vi "获取MPPT状态.vi"(8 "error in (no error)":errorcluster, 11 "MB session in":refnum<class "MB_Master.lvclass">) -> (0 "error out":errorcluster, 1 "结果字符串":string caption="状态", 2 "状态":T1, 3 "MB session out":refnum<class "MB_Master.lvclass">)   [LabVIEW 2016, in "环境动力单元.lvlib"]
uses:
  <vilib>/Plasmionique/MB Master/MB_Master/MB_Master.lvclass
  <vilib>/Plasmionique/MB Master/MB Master.lvlib
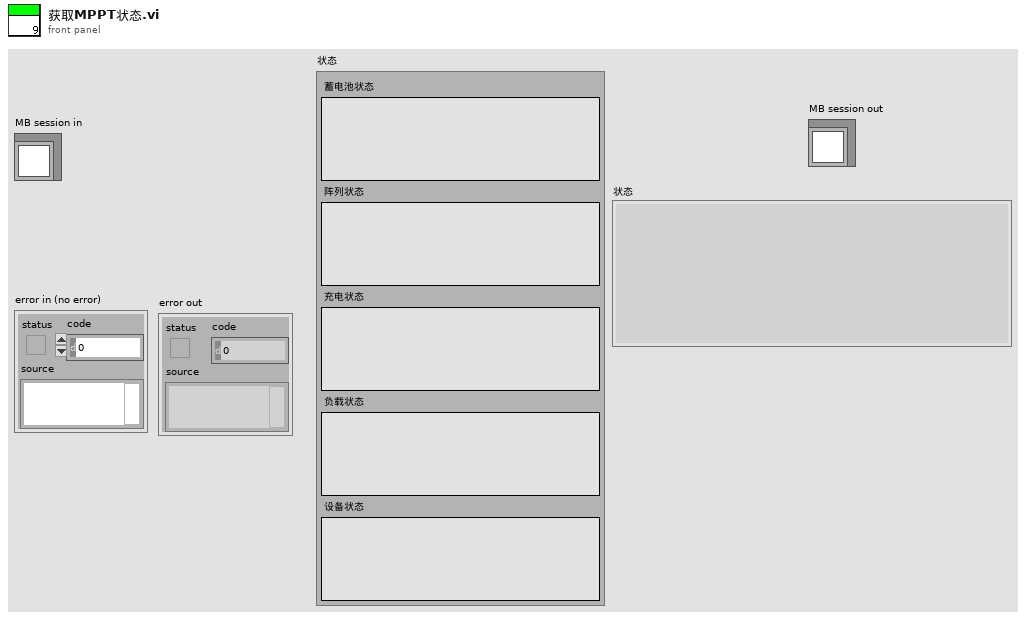
[diagram p1: front panel]
types:
  T1 = cluster{"蓄电池状态":string, "阵列状态":string, "充电状态":string, "负载状态":string, "设备状态":string}
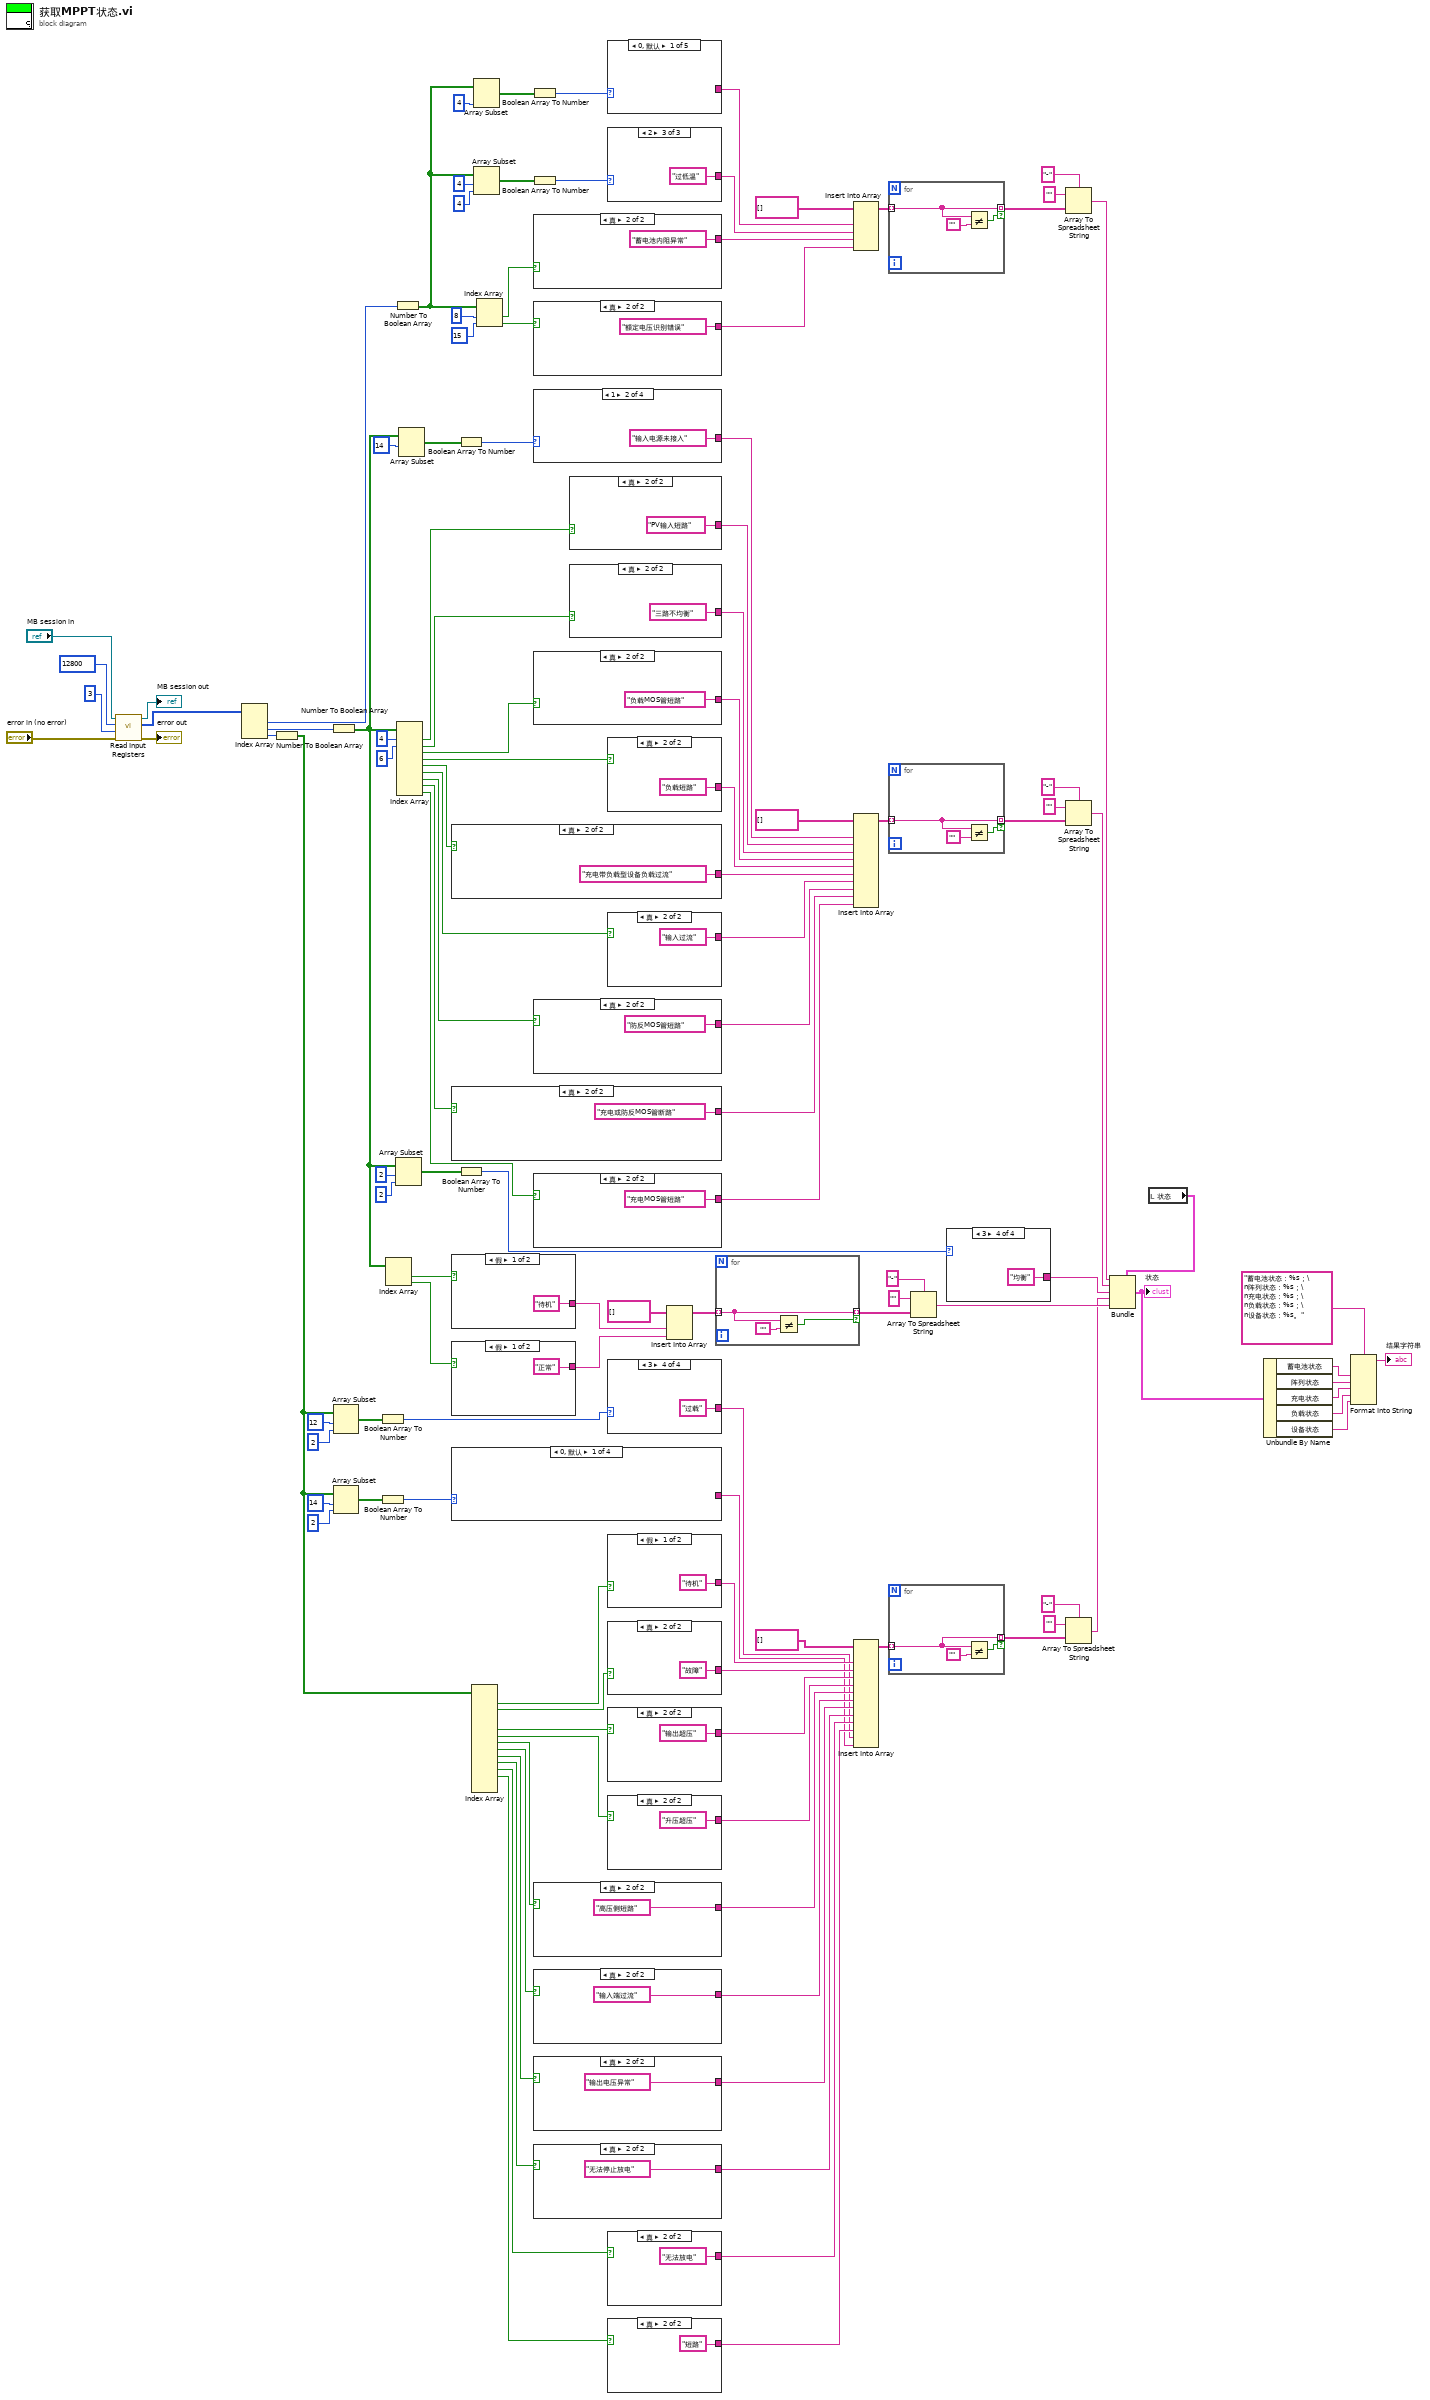
[diagram p0: block diagram]
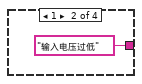
[diagram p2: hidden frame]
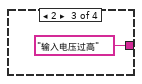
[diagram p3: hidden frame]
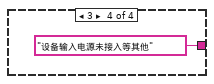
[diagram p4: hidden frame]
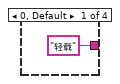
[diagram p5: hidden frame]
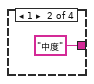
[diagram p6: hidden frame]
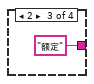
[diagram p7: hidden frame]
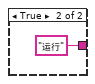
[diagram p17: hidden frame]
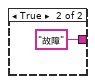
[diagram p18: hidden frame]
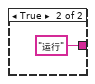
[diagram p19: hidden frame]
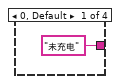
[diagram p20: hidden frame]
diagram:
  n1 = call <vilib>:"Read Input Registers.vi"("error in (no error)"="error in (no error)", "quantity"=u16 3, "starting address"=u16 12800, "MB session in"="MB session in") -> ("error out"=→"error out":errorcluster, "Registers"=w118:u16[], "MB session out"=→"MB session out":refnum<class "MB_Master.lvclass">)  [unwired: 5 in]
  n2 = Index Array(array=w118) -> (element #1=w117:u16, element #2=w95:u16, element #3=w47:u16)  [unwired: 3 in]
  n3 = Number To Boolean Array(number=w47) -> (Boolean array=w21:bool[])
  n4 = Number To Boolean Array(number=w95) -> (Boolean array=w60:bool[])
  n5 = Array Subset(array=w21, index=12 ("索引"), length=2 ("长度")) -> (w27:bool[])
  n6 = Array Subset(array=w21, index=14 ("索引"), length=2 ("长度")) -> (w24:bool[])
  n7 = Boolean Array To Number(Boolean array=w27) -> (number=w26:u32)
  n8 = Boolean Array To Number(Boolean array=w24) -> (number=w25:u32)
  n9 = Index Array(array=w60) -> (element #1=w59:bool, element #2=w58:bool)  [unwired: 2 in]
  n10 = Number To Boolean Array(number=w117) -> (Boolean array=w110:bool[])
  n11 = Array Subset(array=w60, index=2 ("索引"), length=2 ("长度")) -> (w63:bool[])
  n12 = Index Array(array=w60, index #1=4 ("索引"), index #2=6 ("索引")) -> (element #1=w80:bool, element #2=w89:bool, element #3=w88:bool, element #4=w87:bool, element #5=w86:bool, element #6=w85:bool, element #7=w84:bool, element #8=w83:bool, element #9=w82:bool)  [unwired: 7 in]
  n13 = Array Subset(array=w60, index=14 ("索引")) -> (w93:bool[])  [unwired: 1 in]
  n14 = case shown="真" w86 {
    tunnel: [_ "充电带负载型设备负载过流"] -> w70
    frame False {
    }
    frame True {
    }
  }
  n15 = case shown="真" w83 {
    tunnel: [_ "充电或防反MOS管断路"] -> w67
    frame False {
    }
    frame True {
    }
  }
  n16 = case shown="假" w59 {
    tunnel: ["待机" "运行"] -> w50
    frame False {
    }
    frame True {
    }
  }
  n17 = case shown="假" w58 {
    tunnel: ["正常" "故障"] -> w49
    frame False {
    }
    frame True {
    }
  }
  n18 = case shown="0, 默认" w25 {
    tunnel: [_ "输入电压过低" "输入电压过高" "设备输入电源未接入等其他"] -> w10
    frame 0, Default {
    }
    frame 1 {
    }
    frame 2 {
    }
    frame 3 {
    }
  }
  n19 = Boolean Array To Number(Boolean array=w93) -> (number=w92:u32)
  n20 = Boolean Array To Number(Boolean array=w63) -> (number=w62:u32)
  n21 = Index Array(array=w21) -> (element #1=w38:bool, element #2=w39:bool, element #5=w37:bool, element #6=w36:bool, element #7=w35:bool, element #8=w34:bool, element #9=w33:bool, element #10=w32:bool, element #11=w31:bool, element #12=w30:bool)  [unwired: 14 in, 4 out]
  n22 = Array Subset(array=w110, length=4 ("长度")) -> (w115:bool[])  [unwired: 1 in]
  n23 = Array Subset(array=w110, index=4 ("长度"), length=4 ("长度")) -> (w111:bool[])
  n24 = Index Array(array=w110, index #1=8 ("索引"), index #2=15 ("索引")) -> (element #1=w109:bool, element #2=w106:bool)
  n25 = Boolean Array To Number(Boolean array=w115) -> (number=w114:u32)
  n26 = Boolean Array To Number(Boolean array=w111) -> (number=w96:u32)
  n27 = case shown="真" w109 {
    tunnel: [_ "蓄电池内阻异常"] -> w102
    frame False {
    }
    frame True {
    }
  }
  n28 = case shown="真" w106 {
    tunnel: [_ "额定电压识别错误"] -> w101
    frame False {
    }
    frame True {
    }
  }
  n29 = case shown="1" w92 {
    tunnel: [_ "输入电源未接入" "输入电压过高" "输入电压错误"] -> w57
    frame 0, Default {
    }
    frame 1 {
    }
    frame 2 {
    }
    frame 3 {
    }
  }
  n30 = case shown="真" w88 {
    tunnel: [_ "负载MOS管短路"] -> w72
    frame False {
    }
    frame True {
    }
  }
  n31 = case shown="真" w84 {
    tunnel: [_ "防反MOS管短路"] -> w68
    frame False {
    }
    frame True {
    }
  }
  n32 = case shown="真" w82 {
    tunnel: [_ "充电MOS管短路"] -> w66
    frame False {
    }
    frame True {
    }
  }
  n33 = case shown="真" w35 {
    tunnel: [_ "高压侧短路"] -> w18
    frame False {
    }
    frame True {
    }
  }
  n34 = case shown="真" w34 {
    tunnel: [_ "输入端过流"] -> w16
    frame False {
    }
    frame True {
    }
  }
  n35 = case shown="真" w33 {
    tunnel: [_ "输出电压异常"] -> w15
    frame False {
    }
    frame True {
    }
  }
  n36 = case shown="真" w32 {
    tunnel: [_ "无法停止放电"] -> w14
    frame False {
    }
    frame True {
    }
  }
  n37 = case shown="真" w80 {
    tunnel: [_ "PV输入短路"] -> w74
    frame False {
    }
    frame True {
    }
  }
  n38 = case shown="真" w89 {
    tunnel: [_ "三路不均衡"] -> w73
    frame False {
    }
    frame True {
    }
  }
  n39 = case shown="0, 默认" w114 {
    tunnel: [_ "超压" "欠压" "过放" "错误"] -> w105
    frame 0, Default {
    }
    frame 1 {
    }
    frame 2 {
    }
    frame 3 {
    }
    frame 4 {
    }
  }
  n40 = case shown="2" w96 {
    tunnel: [_ "过高温" "过低温"] -> w103
    frame 0, Default {
    }
    frame 1 {
    }
    frame 2 {
    }
  }
  n41 = case shown="真" w87 {
    tunnel: [_ "负载短路"] -> w71
    frame False {
    }
    frame True {
    }
  }
  n42 = case shown="真" w85 {
    tunnel: [_ "输入过流"] -> w69
    frame False {
    }
    frame True {
    }
  }
  n43 = case shown="3" w26 {
    tunnel: ["轻载" "中度" "额定" "过载"] -> w11
    frame 0, Default {
    }
    frame 1 {
    }
    frame 2 {
    }
    frame 3 {
    }
  }
  n44 = case shown="假" w38 {
    tunnel: ["待机" "运行"] -> w45
    frame False {
    }
    frame True {
    }
  }
  n45 = case shown="真" w39 {
    tunnel: [_ "故障"] -> w46
    frame False {
    }
    frame True {
    }
  }
  n46 = case shown="真" w37 {
    tunnel: [_ "输出超压"] -> w20
    frame False {
    }
    frame True {
    }
  }
  n47 = case shown="真" w36 {
    tunnel: [_ "升压超压"] -> w19
    frame False {
    }
    frame True {
    }
  }
  n48 = case shown="真" w31 {
    tunnel: [_ "无法放电"] -> w13
    frame False {
    }
    frame True {
    }
  }
  n49 = case shown="真" w30 {
    tunnel: [_ "短路"] -> w12
    frame False {
    }
    frame True {
    }
  }
  n50 = Insert Into Array(array=string[] [] ("数组"), new element #1=w50, new element #2=w49) -> (w52:string[])  [unwired: 1 in]
  n51 = for {
    tunnel: w52 -> [w168] mode=indexing
    tunnel: [w168] -> w53 mode=indexing if=w167
    n52 = Not Equal?(x=w168, y="") -> (x != y?=w167:bool)
  }
  n53 = Insert Into Array(array=string[] [] ("数组"), new element #1=w105, new element #2=w103, new element #3=w102, new element #4=w101) -> (w100:string[])  [unwired: 1 in]
  n54 = Insert Into Array(array=string[] [] ("数组"), new element #1=w57, new element #2=w74, new element #3=w73, new element #4=w72, new element #5=w71, new element #6=w70, new element #7=w69, new element #8=w68, new element #9=w67, new element #10=w66) -> (w78:string[])  [unwired: 1 in]
  n55 = Insert Into Array(array=string[] [] ("数组"), new element #1=w45, new element #2=w46, new element #3=w20, new element #4=w19, new element #5=w18, new element #6=w16, new element #7=w15, new element #8=w14, new element #9=w13, new element #10=w12, new element #11=w11, new element #12=w10) -> (w43:string[])  [unwired: 1 in]
  n56 = for {
    tunnel: w100 -> [w171] mode=indexing
    tunnel: [w171] -> w99 mode=indexing if=w170
    n57 = Not Equal?(x=w171, y="") -> (x != y?=w170:bool)
  }
  n58 = for {
    tunnel: w78 -> [w174] mode=indexing
    tunnel: [w174] -> w77 mode=indexing if=w173
    n59 = Not Equal?(x=w174, y="") -> (x != y?=w173:bool)
  }
  n60 = for {
    tunnel: w43 -> [w177] mode=indexing
    tunnel: [w177] -> w42 mode=indexing if=w176
    n61 = Not Equal?(x=w177, y="") -> (x != y?=w176:bool)
  }
  n62 = Array To Spreadsheet String(delimiter (Tab)="-" ("分隔符(Tab)"), array=w53, 3:"" ("格式字符串")) -> (spreadsheet string=w48:string)
  n63 = case shown="3" w62 {
    tunnel: ["未充电" "浮充" "提升" "均衡"] -> w61
    frame 0, Default {
    }
    frame 1 {
    }
    frame 2 {
    }
    frame 3 {
    }
  }
  n64 = Array To Spreadsheet String(delimiter (Tab)="-" ("分隔符(Tab)"), array=w99, 3:"" ("格式字符串")) -> (spreadsheet string=w91:string)
  n65 = Array To Spreadsheet String(delimiter (Tab)="-" ("分隔符(Tab)"), array=w77, 3:"" ("格式字符串")) -> (spreadsheet string=w56:string)
  n66 = Array To Spreadsheet String(delimiter (Tab)="-" ("分隔符(Tab)"), array=w42, 3:"" ("格式字符串")) -> (spreadsheet string=w17:string)
  n67 = local read "状态"() -> (w8:T1)
  n68 = Bundle(cluster=w8, "蓄电池状态"=w91, "阵列状态"=w56, "充电状态"=w61, "负载状态"=w17, "设备状态"=w48) -> (w7:T1)
  "状态" <- w7
  n69 = Unbundle By Name(w7) -> ("蓄电池状态"=w6:string, "阵列状态"=w5:string, "充电状态"=w4:string, "负载状态"=w3:string, "设备状态"=w2:string)
  n70 = Format Into String(format string="蓄电池状态：%s；\n阵列状态：%s；\n充电状态：%s；\n负载状态：%s；\n设备状态：%s。" ("格式字符串"), w6, w5, w4, w3, w2) -> (resulting string=→"结果字符串":string)  [unwired: 2 in, 1 out]
